vi "TimeoutCounter.vi"(11 "config in":T1) -> (3 "config out":T1)   [LabVIEW 2017, in "TestPanel.lvlib"]
uses:
  <vilib>/addons/InsightCM/Devices/Shared/Common/TestPanel/TestPanel.lvlib
  <vilib>/addons/InsightCM/Devices/Shared/Common/TestPanel/controls/Configuration.ctl
  <vilib>/addons/InsightCM/Devices/Shared/Common/TestPanel/controls/State.ctl
  <vilib>/addons/InsightCM/MessageBus/Base/controls/IRoutingSource.ctl
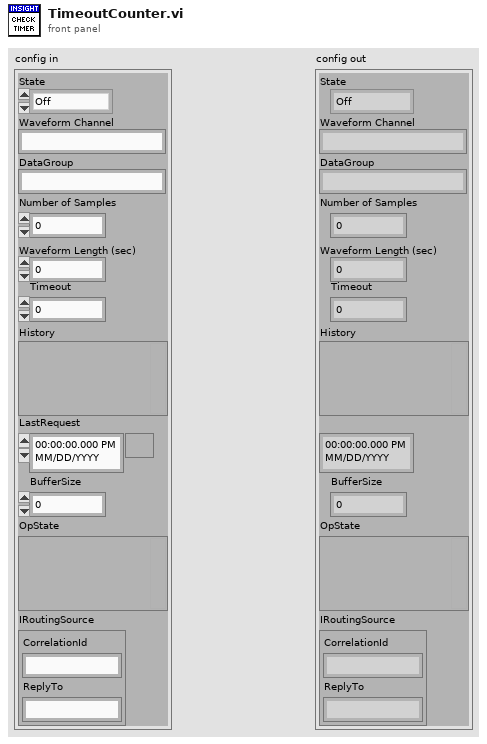
[diagram p1: front panel]
types:
  T1 = typedef "TestPanel.lvlib/Configuration.ctl" = cluster{"State":T2, "Waveform Channel":string, "DataGroup":string, "Number of Samples":i32, "Waveform Length (sec)":dbl, "Timeout":dbl, "History":variant, "LastRequest":timestamp, "BufferSize":i32, "OpState":variant, "IRoutingSource":T3}
  T2 = typedef "TestPanel.lvlib/State.ctl" = enum16{"Off", "On", "PendingValues", "PendingDataSet"}
  T3 = typedef "IRoutingSource.ctl" = cluster{"CorrelationId":string, "ReplyTo":string}
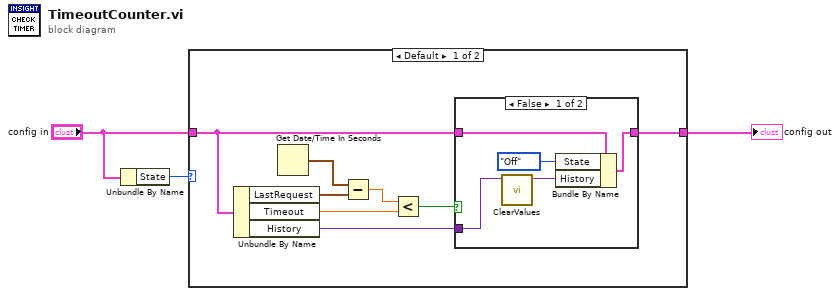
[diagram p0: block diagram]
diagram:
  n1 = Unbundle By Name("config in") -> ("State"=w3:T2)
  n2 = case shown="Default" w3 {
    tunnel: "config in" -> [w11 w18]
    tunnel: [w10 w18] -> w1
    frame Default {
      n3 = Unbundle By Name(w11) -> ("LastRequest"=w8:timestamp, "Timeout"=w6:dbl, "History"=w4:variant)
      n4 = Get Date/Time In Seconds() -> (seconds since 1Jan1904=w9:timestamp)
      n5 = Subtract(x=w9, y=w8) -> (x-y=w7:dbl)
      n6 = Less?(x=w7, y=w6) -> (x < y?=w5:bool)
      n7 = case shown="False" w5 {
        tunnel: w11 -> [w16 w17]
        tunnel: [w15 w17] -> w10
        tunnel: w4 -> [w13 _]
        frame False {
          n8 = call <vilib>:"ClearValues.vi"("history in"=w13) -> ("history out"=w12:variant)  [unwired: 9 in, 1 out]
          n9 = Bundle By Name(cluster=w16, "State"=State."Off", "History"=w12) -> (w15:T1)
        }
        frame True {
        }
      }
    }
    frame "Off" {
    }
  }
  "config out" <- w1
